vi "LeerArchivoConfiguracion.vi"(8 "error in":errorcluster, 11 "Prueba31 in":refnum<class "Prueba33.lvclass">) -> (0 "error out":errorcluster, 3 "Prueba31 out":refnum<class "Prueba33.lvclass">)   [LabVIEW 2019, in "Prueba33.lvclass"]
uses:
  Prueba33.lvclass
  Prueba33.lvclass/Prueba33.ctl
  <vilib>/Utility/config.llb/Read Key (Boolean).vi
  <vilib>/Utility/config.llb/Read Key (String).vi
  <vilib>/Utility/config.llb/NI_LVConfig.lvlib
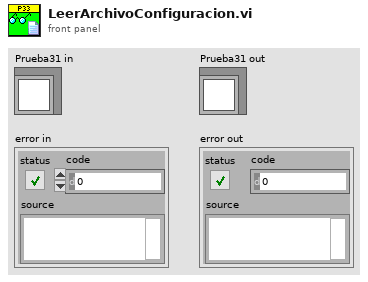
[diagram p1: front panel]
types:
  T1 = typedef "NI_LVConfig.lvlib/Config Data RefNum.ctl" = refnum<k1>
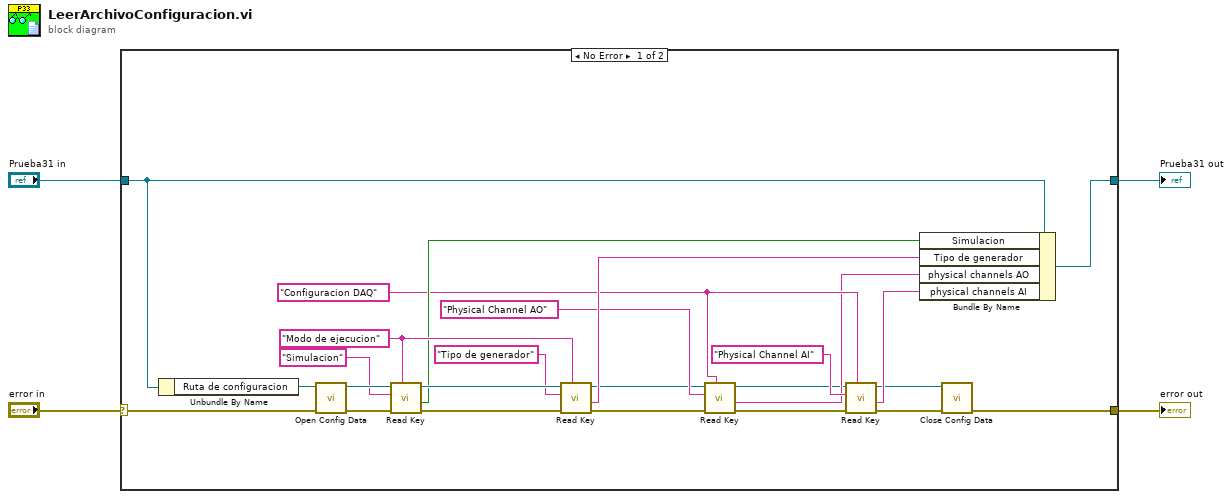
[diagram p0: block diagram]
diagram:
  n1 = case shown="No Error" "error in" {
    selector: "error in" -> [w29 w30]
    tunnel: [w18 w30] -> w2
    tunnel: [w17 w31] -> w4
    tunnel: "Prueba31 in" -> [w16 w31]
    frame No Error {
      w13 = "Configuracion DAQ" ("section")
      w23 = "Modo de ejecucion" ("section")
      n2 = Unbundle By Name(w16) -> ("Ruta de configuracion"=w28:path)
      n3 = call <vilib>:"Open Config Data.vi"("error in (no error)"=w29, "configuration file path"=w28) -> ("error out"=w27:errorcluster, "refnum"=w26:T1)  [unwired: 7 in, 1 out]
      n4 = call-poly <vilib>:"Read Key.vi"("section"=w23, "error in (no error)"=w27, "key"="Simulacion", "refnum"=w26) -> ("error out"=w22:errorcluster, "value"=w21:bool, "refnum out"=w24:T1)  [unwired: 4 in, 1 out]
      n5 = call-poly <vilib>:"Read Key.vi"("section"=w23, "error in (no error)"=w22, "key"="Tipo de generador", "refnum"=w24) -> ("error out"=w7:errorcluster, "value"=w19:string, "refnum out"=w10:T1)  [unwired: 4 in, 1 out]
      n6 = call-poly <vilib>:"Read Key.vi"("section"=w13, "error in (no error)"=w7, "key"="Physical Channel AO", "refnum"=w10) -> ("error out"=w6:errorcluster, "value"=w12:string, "refnum out"=w9:T1)  [unwired: 4 in, 1 out]
      n7 = call-poly <vilib>:"Read Key.vi"("section"=w13, "error in (no error)"=w6, "key"="Physical Channel AI", "refnum"=w9) -> ("error out"=w5:errorcluster, "value"=w11:string, "refnum out"=w8:T1)  [unwired: 4 in, 1 out]
      n8 = Bundle By Name(cluster=w16, "Simulacion"=w21, "Tipo de generador"=w19, "physical channels AO"=w12, "physical channels AI"=w11) -> (w17:refnum<class "Prueba33.lvclass">)
      n9 = call <vilib>:"Close Config Data.vi"("error in (no error)"=w5, "refnum"=w8) -> ("error out"=w18:errorcluster)  [unwired: 8 in, 1 out]
    }
    frame Error {
    }
  }
  "Prueba31 out" <- w4
  "error out" <- w2
